vi "FGV SysLog PC.vi"(6 "Aktion":T3, 7 "SysLogLevel":u32, 8 "Fehler (in)":errorcluster caption="Fehler in", 9 "Main History Button Referenz in":refnum<vi>, 10 "Syslog Anforderung":bool, 11 "Cluster  (in)":T2) -> (0 "Fehler (out)":errorcluster caption="Fehlerausgang", 1 "Main History Button Referenz out":refnum<vi>, 2 "Syslog Anforderung":bool, 3 "Anzeige Cluster":T1, 4 "Fehler out":errorcluster[](array[cluster]))   [LabVIEW 2015, in "SysLog.lvlib"]
doc: "FGV zum Sammeln von Error Meldungen die mit den Betriebsdaten in eine\n#ErrLogHistory geschreiben werden \ninitialisieren ... erzeugt ein Array (auch zum Zurücksetzen)\nspeichern ... zum Hinzufügen einer neuen Fehlermeldung\nlesen ... zum auslesen des Arrays \n\nriw 8.6.2018"
uses:
  SysLog.lvlib
  Aktionen FGV SysLog.ctl
  <vilib>/regexp/Match Regular Expression.xnode
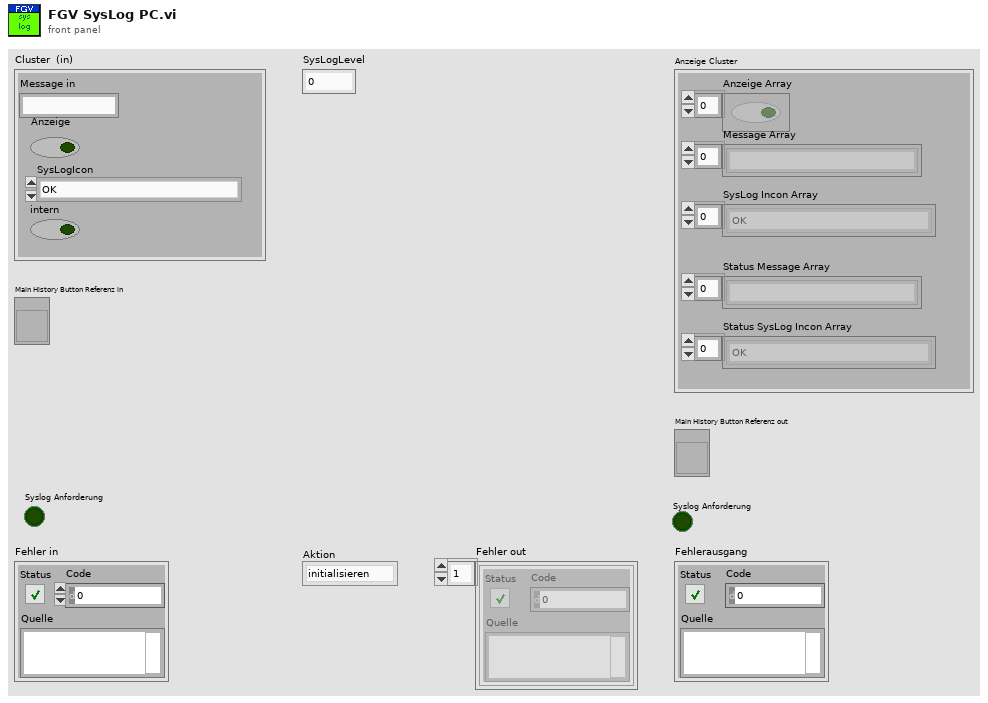
[diagram p1: front panel]
types:
  T1 = cluster{"Anzeige Array":bool[], "Message Array":string[], "SysLog Incon Array":enum16{"OK", "Warnung", "Fehler"}[], "Status Message Array":string[], "Status SysLog Incon Array":enum16{"OK", "Warnung", "Fehler"}[]}
  T2 = cluster{"Message in":string, "Anzeige":bool, "SysLogIcon":enum16{"OK", "Warnung", "Fehler"}, "intern":bool}
  T3 = typedef "SysLog.lvlib/Aktionen FGV SysLog.ctl" = enum16{"initialisieren", "lesen", "schreiben", "history button ref", "Syslog_Anforderung"}
  T4 = cluster{bool[], string[], enum16{"OK", "Warnung", "Fehler"}[], string[], enum16{"OK", "Warnung", "Fehler"}[]}
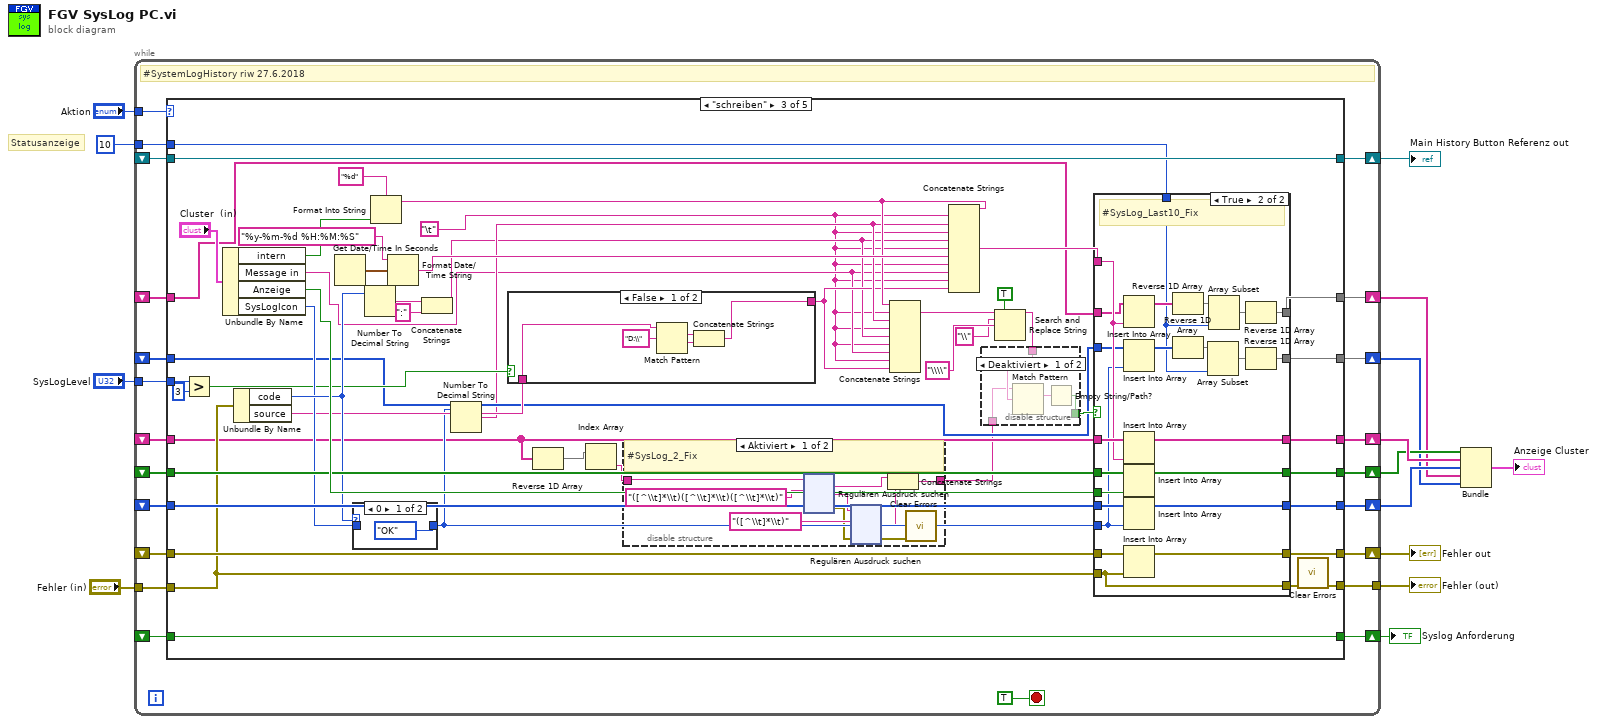
[diagram p0: block diagram]
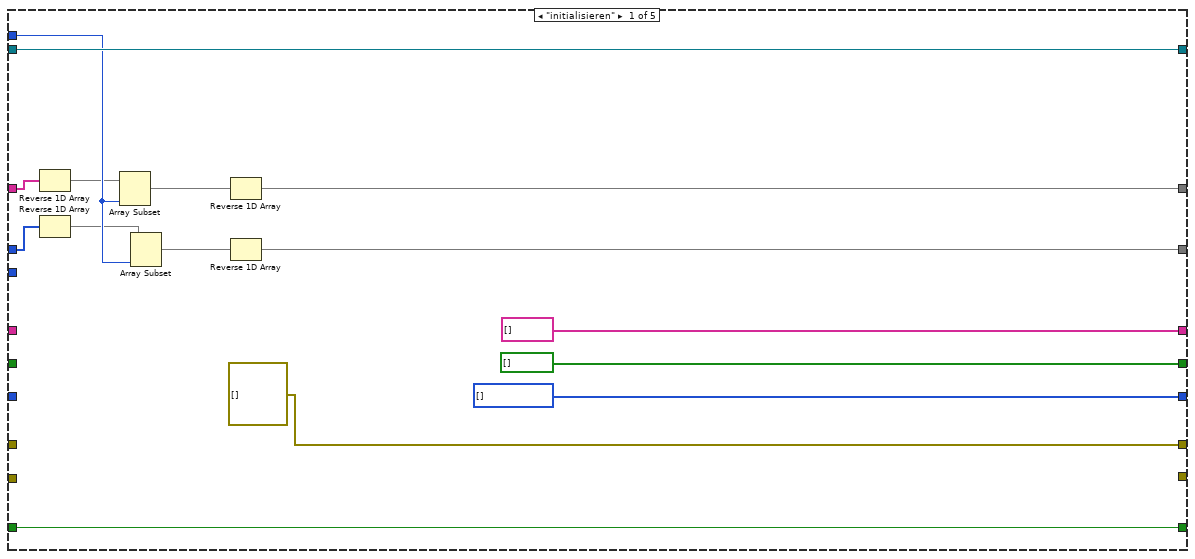
[diagram p2: hidden frame]
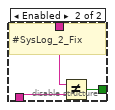
[diagram p4: hidden frame]
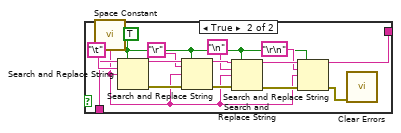
[diagram p7: hidden frame]
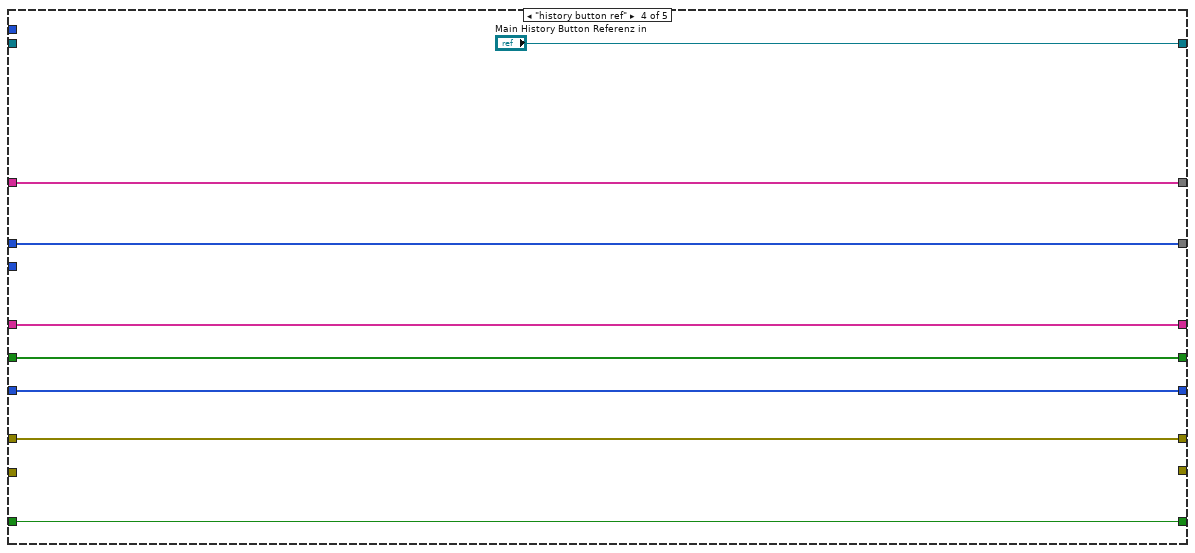
[diagram p9: hidden frame]
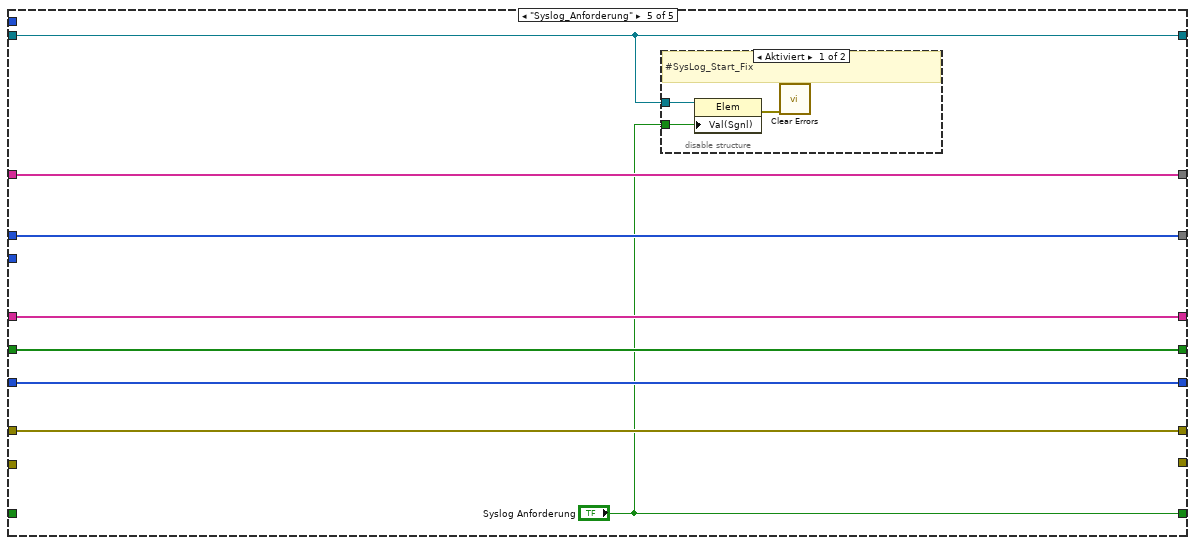
[diagram p10: hidden frame]
diagram:
  # "Statusanzeige"
  n1 = while {
    tunnel: "Aktion" -> [w35]
    shift-right: [w33] -> w13
    shift-left: _ -> [w34]
    shift-right: [w32] -> w6
    shift-left: _ -> [w31]
    tunnel: [w30] -> w12
    shift-right: [w29] -> w8
    shift-left: _ -> [w28]
    shift-right: [w27] -> w7
    shift-left: _ -> [w26]
    tunnel: "SysLogLevel" -> [w25]
    tunnel: "Fehler (in)" -> [w24]
    shift-right: [w23] -> w9
    shift-left: _ -> [w22]
    shift-right: [w21] -> w4
    shift-left: _ -> [w20]
    shift-right: [w19] -> w3
    shift-left: _ -> [w18]
    tunnel: 10 ("Länge") -> [w17]
    shift-right: [w16] -> w1
    shift-left: _ -> [w15]
    stop <- TRUE stop-if-true
    # "#SystemLogHistory riw 27.6.2018"
    n2 = case shown="\"schreiben\"" w35 {
      tunnel: w34 -> [_ w59 w108 w414 w422]
      tunnel: [errorcluster[] [] ("Fehler out") w59 w107 w414 w422] -> w33
      tunnel: [w50 w58 w80 w413 w421] -> w32
      tunnel: w31 -> [_ w58 w109 w413 w421]
      tunnel: [_ _ w106 _ _] -> w30
      tunnel: [string[] [] w57 w81 w412 w420] -> w29
      tunnel: w28 -> [_ w57 w71 w412 w420]
      tunnel: [bool[] [] w56 w99 w411 w419] -> w27
      tunnel: w26 -> [_ w56 w98 w411 w419]
      tunnel: w25 -> [_ _ w92 _ _]
      tunnel: w24 -> [_ _ w73 _ _]
      tunnel: [w47 w55 w82 "Main History Button Referenz in" w416] -> w23
      tunnel: w22 -> [w47 w55 w82 _ w416]
      tunnel: [w39 w54 w75 w409 w418] -> w21
      tunnel: w20 -> [w43 w54 w78 w409 w418]
      tunnel: [w38 w53 w74 w408 w417] -> w19
      tunnel: w18 -> [w42 w53 w77 w408 w417]
      tunnel: w17 -> [w44 _ w76 _ _]
      tunnel: [w37 w52 w72 w407 "Syslog Anforderung"] -> w16
      tunnel: w15 -> [w37 w52 w72 w407 _]
      frame "initialisieren" {
        w50 = enum16{"OK", "Warnung", "Fehler"}[] [] items=["OK", "Warnung", "Fehler"]
        n3 = Reverse 1D Array(array=w43) -> (reversed array=w41:string[])
        n4 = Reverse 1D Array(array=w42) -> (reversed array=w40:enum16{"OK", "Warnung", "Fehler"}[])
        n5 = Array Subset(array=w41, length=w44) -> (w46:string[])  [unwired: 1 in]
        n6 = Array Subset(array=w40, length=w44) -> (w45:enum16{"OK", "Warnung", "Fehler"}[])  [unwired: 1 in]
        n7 = Reverse 1D Array(array=w46) -> (reversed array=w39:string[])
        n8 = Reverse 1D Array(array=w45) -> (reversed array=w38:enum16{"OK", "Warnung", "Fehler"}[])
      }
      frame "lesen", Default {
      }
      frame "schreiben" {
        w61 = "\t"
        n9 = Greater?(x=w92, y=u32 3) -> (0:w90:bool)
        n10 = Unbundle By Name("Cluster  (in)") -> ("intern"=w83:bool, "Message in"=w62:string, "Anzeige"=w100:bool, "SysLogIcon"=w96:enum16{"OK", "Warnung", "Fehler"})
        n11 = Unbundle By Name(w73) -> ("code"=w97:i32, "source"=w95:string)
        n12 = Get Date/Time In Seconds() -> (seconds since 1Jan1904=w105:timestamp)
        n13 = case shown="0" w97 {
          tunnel: [enum16{"OK", "Warnung", "Fehler"}."OK" ("SysLogIcon") w406] -> w93
          tunnel: w96 -> [_ w406]
          frame 0 {
          }
          frame Default {
          }
        }
        n14 = Number To Decimal String(number=w97) -> (decimal integer string=w102:string)  [unwired: 1 in]
        n15 = Format Into String(format string="%d" ("Format-String"), w83) -> (resulting string=w66:string)  [unwired: 2 in, 1 out]
        n16 = Format Date/Time String(time format string (%c)="%y-%m-%d %H:%M:%S" ("Zeitformatierungs-String (%c)"), seconds (now)=w105) -> (date/time string=w103:string)  [unwired: 1 in]
        n17 = Concatenate Strings(w102, ":") -> (w63:string)
        n18 = Number To Decimal String(number=w93) -> (decimal integer string=w65:string)  [unwired: 1 in]
        n19 = case shown="False" w90 {
          tunnel: w95 -> [w386 w393]
          tunnel: [w385 w391] -> w64
          frame False {
            n20 = Match Pattern(string=w386, regular expression="D:\\") -> (match substring=w388:string, after substring=w387:string)  [unwired: 1 in, 2 out]
            n21 = Concatenate Strings(w388, w387) -> (w385:string)
          }
          frame True {
            w390 = TRUE ("Alle ersetzen? (F)")
            n22 = call <vilib>:"Space Constant.vi"() -> ("String"=w392:string)
            n23 = Search and Replace String(replace all?=w390, input string=w393, search string="\t", replace string=w392) -> (result string=w403:string, error out=w402:errorcluster)  [unwired: 4 in, 2 out]
            n24 = Search and Replace String(replace all?=w390, input string=w403, search string="\r", replace string=w392, error in=w402) -> (result string=w400:string, error out=w397:errorcluster)  [unwired: 3 in, 2 out]
            n25 = Search and Replace String(replace all?=w390, input string=w400, search string="\n", replace string=w392, error in=w397) -> (result string=w398:string, error out=w396:errorcluster)  [unwired: 3 in, 2 out]
            n26 = Search and Replace String(replace all?=w390, input string=w398, search string="\r\n", replace string=w392, error in=w396) -> (result string=w391:string, error out=w395:errorcluster)  [unwired: 3 in, 2 out]
            n27 = call <vilib>:"Clear Errors.vi"("error in (no error)"=w395) -> ()  [unwired: 5 in, 2 out]
          }
        }
        n28 = Reverse 1D Array(array=w71) -> (reversed array=w70:string[])
        n29 = Index Array(array=w70) -> (element=w69:string)  [unwired: 1 in]
        n30 = disable-structure shown="Aktiviert" {
          disable-tunnel: w69 -> [w117 w354]
          disable-tunnel: [w119 w354] -> w68
          frame Enabled {
            # "#SysLog_2_Fix"
            n31 = xnode "Regulären Ausdruck suchen"("Eingangs-String"=w117, "Regulärer Ausdruck"="([^\\t]*\\t)([^\\t]*\\t)([^\\t]*\\t)") -> ("Komplette Übereinstimmung"=w118:string, "Nach Übereinstimmung"=w124:string, "Fehler (Ausgang)"=w122:errorcluster)  [unwired: 4 in, 2 out]
            n32 = xnode "Regulären Ausdruck suchen"("Eingangs-String"=w124, "Regulärer Ausdruck"="([^\\t]*\\t)", "Fehler (Eingang)"=w122) -> ("Nach Übereinstimmung"=w120:string, "Fehler (Ausgang)"=w121:errorcluster)  [unwired: 3 in, 3 out]
            n33 = Concatenate Strings(w118, w120) -> (w119:string)
            n34 = call <vilib>:"Clear Errors.vi"("error in (no error)"=w121) -> ()  [unwired: 5 in, 2 out]
          }
          frame Disabled {
          }
        }
        n35 = Concatenate Strings(w66, w61, w65, w61, w63, w61, w62, w61, w64) -> (w67:string)
        n36 = Concatenate Strings(w66, w61, w65, w61, w63, w61, w103, w61, w62, w61, w64) -> (w79:string)
        n37 = Search and Replace String(replace all?=TRUE ("Alle ersetzen? (F)"), input string=w67, search string="\\", replace string="\\\\") -> (result string=w60:string)  [unwired: 4 in, 3 out]
        n38 = disable-structure shown="Deaktiviert" {
          disable-tunnel: [w112 w114] -> w89
          disable-tunnel: w60 -> [w111 w115]
          disable-tunnel: w68 -> [w110 w116]
          frame Disabled {
            n39 = Match Pattern(string=w110, regular expression=w111) -> (match substring=w113:string)  [unwired: 1 in, 3 out]
            n40 = Empty String/Path?(string/path=w113) -> (empty?=w112:bool)
          }
          frame Enabled {
            # "#SysLog_2_Fix"
            n41 = Not Equal?(x=w115, y=w116) -> (x != y?=w114:bool)
          }
        }
        n42 = case shown="True" w89 {
          tunnel: w109 -> [w359 w384]
          tunnel: [w359 w383] -> w80
          tunnel: w108 -> [w358 w382]
          tunnel: [w358 w381] -> w107
          tunnel: w79 -> [_ w374]
          tunnel: [w361 w380] -> w81
          tunnel: w100 -> [_ w379]
          tunnel: [w360 w378] -> w99
          tunnel: w71 -> [w361 w377]
          tunnel: w98 -> [w360 w376]
          tunnel: w93 -> [_ w373]
          tunnel: w73 -> [w357 w375]
          tunnel: [w357 w375] -> w88
          tunnel: w78 -> [w356 w372]
          tunnel: w77 -> [w355 w371]
          tunnel: w76 -> [_ w368]
          tunnel: [w356 w364] -> w75
          tunnel: [w355 w362] -> w74
          frame False {
            # "nie 2 gleiche"
          }
          frame True {
            # "#SysLog_Last10_Fix"
            n43 = Insert Into Array(array=w372, new element=w374) -> (w370:string[])  [unwired: 1 in]
            n44 = Insert Into Array(array=w371, new element=w373) -> (w369:enum16{"OK", "Warnung", "Fehler"}[])  [unwired: 1 in]
            n45 = Insert Into Array(array=w377, new element=w374) -> (w380:string[])  [unwired: 1 in]
            n46 = Insert Into Array(array=w376, new element=w379) -> (w378:bool[])  [unwired: 1 in]
            n47 = Insert Into Array(array=w384, new element=w373) -> (w383:enum16{"OK", "Warnung", "Fehler"}[])  [unwired: 1 in]
            n48 = Insert Into Array(array=w382, new element=w375) -> (w381:errorcluster[])  [unwired: 1 in]
            n49 = Reverse 1D Array(array=w370) -> (reversed array=w365:string[])
            n50 = Reverse 1D Array(array=w369) -> (reversed array=w363:enum16{"OK", "Warnung", "Fehler"}[])
            n51 = Array Subset(array=w363, length=w368) -> (w366:enum16{"OK", "Warnung", "Fehler"}[])  [unwired: 1 in]
            n52 = Array Subset(array=w365, length=w368) -> (w367:string[])  [unwired: 1 in]
            n53 = Reverse 1D Array(array=w367) -> (reversed array=w364:string[])
            n54 = Reverse 1D Array(array=w366) -> (reversed array=w362:enum16{"OK", "Warnung", "Fehler"}[])
          }
        }
        n55 = call <vilib>:"Clear Errors.vi"("error in (no error)"=w88) -> ("error out"=w106:errorcluster)  [unwired: 5 in, 1 out]
      }
      frame "history button ref" {
      }
      frame "Syslog_Anforderung" {
        n56 = disable-structure shown="Aktiviert" {
          disable-tunnel: "Syslog Anforderung" -> [w424 _]
          disable-tunnel: w416 -> [w423 _]
          frame Enabled {
            # "#SysLog_Start_Fix"
            n57 = property class="Elem"(reference=w423, "Val(Sgnl)"=w424) -> (error out=w425:errorcluster)  [unwired: 1 in, 1 out]
            n58 = call <vilib>:"Clear Errors.vi"("error in (no error)"=w425) -> ()  [unwired: 5 in, 2 out]
          }
          frame Disabled {
          }
        }
      }
    }
  }
  "Fehler out" <- w13
  "Fehler (out)" <- w12
  "Main History Button Referenz out" <- w9
  "Syslog Anforderung" <- w1
  n59 = Bundle(w7, w8, w6, w4, w3) -> (→"Anzeige Cluster":T4)  [unwired: 1 in]
